vi "pmu_Write Time .vi"(8 "error in (no error)":errorcluster, 9 "time quality":u8, 10 "time stamp":timestamp, 11 "system info in":refnum<class "PMU System Info.lvclass">) -> (0 "error out":errorcluster, 3 "system info out":refnum<class "PMU System Info.lvclass">)   [LabVIEW 2011, in "NI_EP_PMU.lvlib" / "PMU System Info.lvclass"]
uses:
  <vilib>/addons/Electrical Power/PMU/Common/Classes/PMU System Info/PMU System Info.lvclass
  <vilib>/addons/Electrical Power/PMU/Common/Controls/pmu_Time&Quality.ctl
  <vilib>/addons/Electrical Power/PMU/Common/Classes/PMU System Info/PMU System Info.lvclass/PMU System Info.ctl
  <vilib>/addons/Electrical Power/PMU/NI_EP_PMU.lvlib
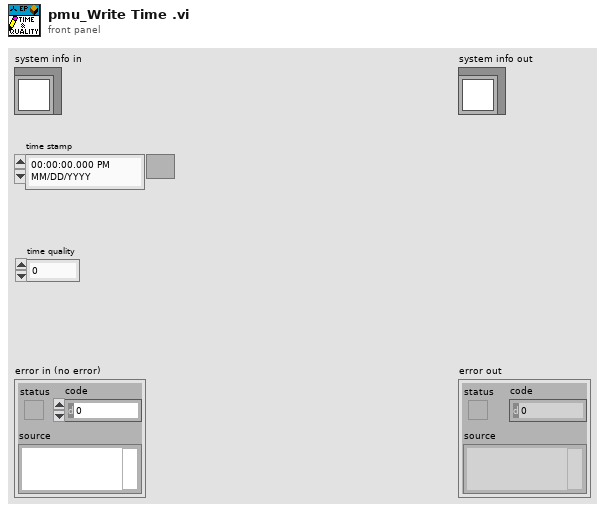
[diagram p1: front panel]
types:
  T1 = typedef "NI_EP_PMU.lvlib/pmu_Time&Quality.ctl" = cluster{"time stamp":timestamp, "time quality":u8}
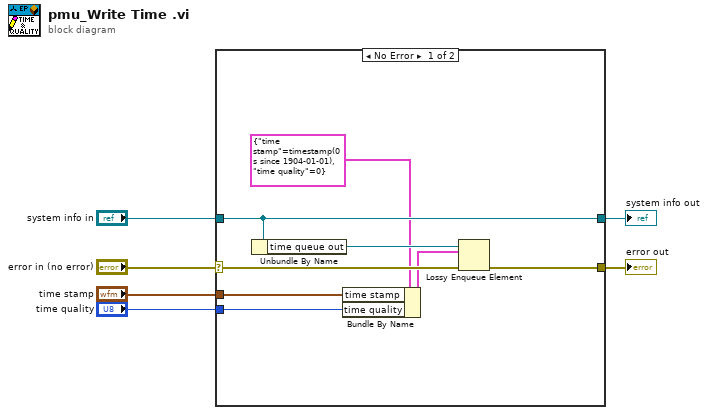
[diagram p0: block diagram]
diagram:
  n1 = case shown="No Error" "error in (no error)" {
    selector: "error in (no error)" -> [w11 w15]
    tunnel: [w10 w15] -> w5
    tunnel: [w9 w16] -> w3
    tunnel: "system info in" -> [w9 w16]
    tunnel: "time stamp" -> [w13 _]
    tunnel: "time quality" -> [w12 _]
    frame No Error {
      n2 = Unbundle By Name(w9) -> ("time queue out"=w14:refnum<queue>)
      n3 = Bundle By Name(cluster=T1 {"time stamp"=timestamp(0 s since 1904-01-01), "time quality"=0} ("Time"), "time stamp"=w13, "time quality"=w12) -> (w7:T1)
      n4 = Lossy Enqueue Element(queue=w14, element=w7, error in (no error)=w11) -> (error out=w10:errorcluster)  [unwired: 3 out]
    }
    frame Error {
    }
  }
  "error out" <- w5
  "system info out" <- w3
